vi "sub_joy analog input.vi"(5 "上限":dbl, 7 "下限":dbl, 9 "lock输入奇偶":dbl, 10 "x":i32, 11 "Displacement":dbl) -> (0 "lock dis.":bool, 1 "x state":i32)   [LabVIEW 2015]
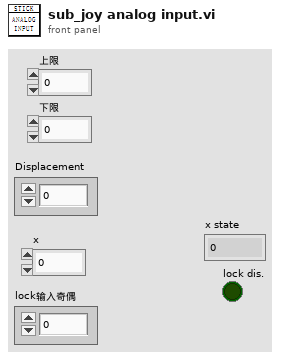
[diagram p1: front panel]
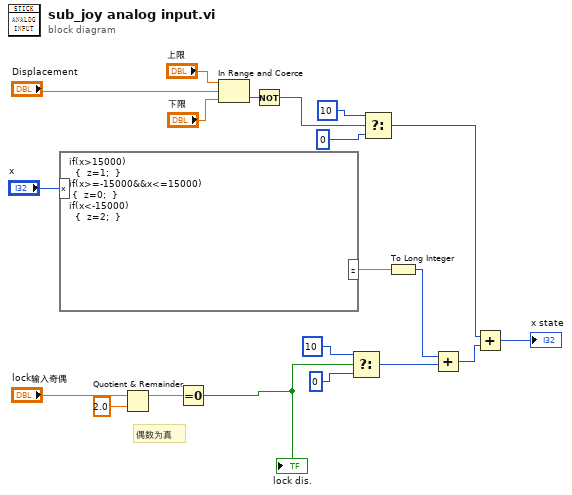
[diagram p0: block diagram]
diagram:
  # "偶数为真"
  n1 = formula code="if(x>15000)\n  {  z=1;  }\nif(x>=-15000&&x<=15000)\n {  z=0;  }\nif(x<-15000)\n  {  z=2;  }"("x"="x") -> ("z"=w19:dbl)
  n2 = Quotient & Remainder(x="lock输入奇偶", y=2.0) -> (x-y*floor(x/y)=w13:dbl)  [unwired: 1 out]
  n3 = Equal To 0?(x=w13) -> (x = 0?=w12:bool)
  "lock dis." <- w12
  n4 = In Range and Coerce(upper limit="上限", x="Displacement", lower limit="下限") -> (In Range?=w2:bool)  [unwired: 1 out]
  n5 = Not(x=w2) -> (.not. x?=w1:bool)
  n6 = Select(t=10 ("32位整型"), s=w12, f=0 ("32位整型")) -> (s? t:f=w17:i32)
  n7 = Select(t=10 ("32位整型"), s=w1, f=0 ("32位整型")) -> (s? t:f=w5:i32)
  n8 = To Long Integer(number=w19) -> (32bit integer=w18:i32)
  n9 = Add(x=w18, y=w17) -> (x+y=w6:i32)
  n10 = Add(x=w5, y=w6) -> (x+y=→"x state":i32)
